vi "Create Rock.vi"(0 "Pyroclastic Rock Shape":T1) -> (1 "Rock Color":u32(colorbox), 2 "Rock":u32[][](array[colorbox]))   [LabVIEW 2020, in "AoC 2022.lvlib"]
uses:
  AoC 2022.lvlib
  Pyroclastic Rock Shape.ctl
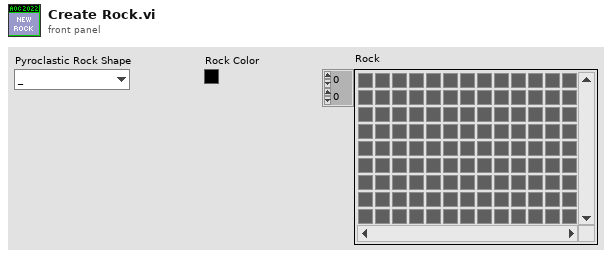
[diagram p1: front panel]
types:
  T1 = typedef "AoC 2022.lvlib/Pyroclastic Rock Shape.ctl" = enum16{"_", "+", "_|", "|", "."}
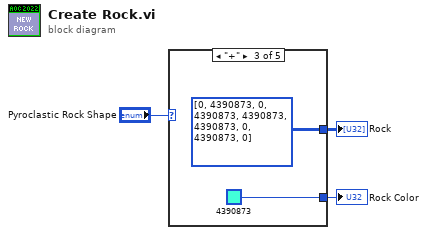
[diagram p0: block diagram]
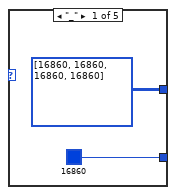
[diagram p2: hidden frame]
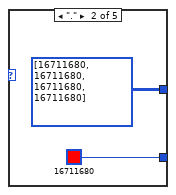
[diagram p3: hidden frame]
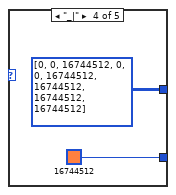
[diagram p4: hidden frame]
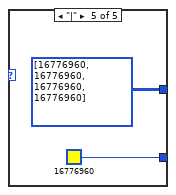
[diagram p5: hidden frame]
diagram:
  n1 = case shown="\"+\"" "Pyroclastic Rock Shape" {
    tunnel: [u32[][] [[16860, 16860, 16860, 16860]] u32[][] [[16711680, 16711680], [16711680, 16711680]] u32[][] [[0, 4390873, 0], [4390873, 4390873, 4390873], [0, 4390873, 0]] u32[][] [[0, 0, 16744512], [0, 0, 16744512], [16744512, 16744512, 16744512]] u32[][] [[16776960], [16776960], [16776960], [16776960]]] -> w3
    tunnel: [u32 16860 ("Color") u32 16711680 ("Color") u32 4390873 ("Color") u32 16744512 ("Color") u32 16776960 ("Color")] -> w1
    frame "_" {
    }
    frame "." {
    }
    frame "+" {
    }
    frame "_|" {
    }
    frame "|" {
    }
  }
  "Rock" <- w3
  "Rock Color" <- w1
